vi "StateMachineEvenButton.vi"() -> ()   [LabVIEW 2014]
panel:
  out "State":enum16{"IDLE", "Play", "Stop", "Init"}(ring)
  in  "Pause":bool
  in  "Start":bool
  in  "Stop":bool
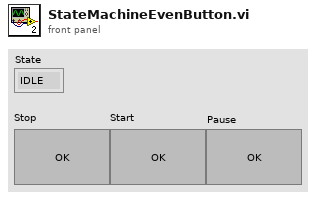
[diagram p1: front panel]
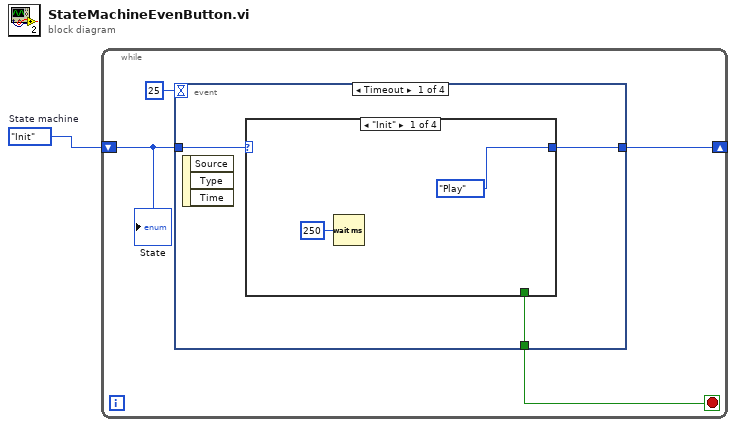
[diagram p0: block diagram]
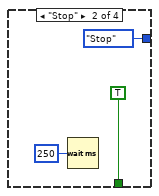
[diagram p2: hidden frame]
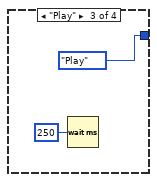
[diagram p3: hidden frame]
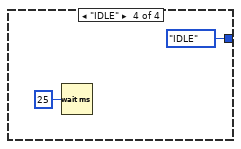
[diagram p4: hidden frame]
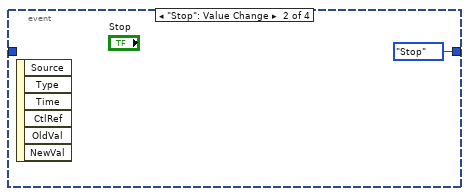
[diagram p5: hidden frame]
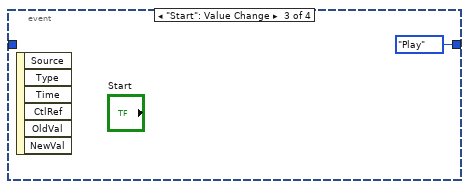
[diagram p6: hidden frame]
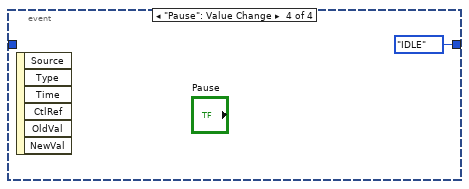
[diagram p7: hidden frame]
diagram:
  w1 = enum16{"IDLE", "Play", "Stop", "Init"}."Init"  # State machine
  n1 = while {
    shift-right: [w3] -> _
    shift-left: w1 -> [w4]
    stop <- w2 stop-if-true
    n2 = event shown="[0] Timeout" {
      selector: _ -> [_ _ _ _]
      dyn-events: _ -> [_ _ _ _]
      timeout: 25 -> [_ _ _ _]
      tunnel: w4 -> [w8 _ _ _]
      tunnel: [w7 enum16{"IDLE", "Play", "Stop", "Init"}."Stop" ("Enum") enum16{"IDLE", "Play", "Stop", "Init"}."Play" ("Enum") enum16{"IDLE", "Play", "Stop", "Init"}."IDLE" ("Enum")] -> w3
      tunnel: [w6 _ _ _] -> w2
      event Timeout {
        n3 = event-data() -> ()  [unwired: 1 in, 3 out]
        n4 = case shown="\"Init\"" w8 {
          tunnel: [enum16{"IDLE", "Play", "Stop", "Init"}."Play" ("Enum") enum16{"IDLE", "Play", "Stop", "Init"}."Stop" ("Enum") enum16{"IDLE", "Play", "Stop", "Init"}."Play" ("Enum") enum16{"IDLE", "Play", "Stop", "Init"}."IDLE" ("Enum")] -> w7
          tunnel: [_ TRUE _ _] -> w6
          frame "Init" {
            n5 = Wait (ms)(milliseconds to wait=u32 250) -> ()  [unwired: 1 out]
          }
          frame "Stop" {
            n6 = Wait (ms)(milliseconds to wait=u32 250) -> ()  [unwired: 1 out]
          }
          frame "Play" {
            n7 = Wait (ms)(milliseconds to wait=u32 250) -> ()  [unwired: 1 out]
          }
          frame "IDLE" {
            n8 = Wait (ms)(milliseconds to wait=u32 25) -> ()  [unwired: 1 out]
          }
        }
      }
      event "Stop": Value Change {
        n9 = event-data() -> ()  [unwired: 1 in, 6 out]
      }
      event "Start": Value Change {
        n10 = event-data() -> ()  [unwired: 1 in, 6 out]
      }
      event "Pause": Value Change {
        n11 = event-data() -> ()  [unwired: 1 in, 6 out]
      }
    }
    "State" <- w4
  }
